vi "Test ClonSubpanel API.vi"() -> ()   [LabVIEW 2024]
doc: "ClonSubpanel API Tester."
uses:
  <vilib>/Utility/error.llb/DialogType.ctl
  ClonSubpanel.lvlib
panel:
  in  "Remove FP from Subpanel":bool
  in  "Draw FP in Supbpanel 2":bool
  in  "Draw FP in Supbpanel 1":bool
  out "last error":errorcluster
  in  "Show Diagram on Init":bool
  in  "Run as Singleton?":bool
  in  "Show Block Diagram":bool
  in  "Refresh Modules":bool
  out "Active Modules":string[](array[string])
  in  "Stop Module":bool
  in  "Select Module":i32(ring)=-1 caption="Select Module\nTo send Request to" items=["All"=-1]
  in  "Run New Module":bool
  in  "Hide Module Panel":bool
  in  "Show Module Panel":bool
  out "Status":string
  # "This VI tests the API for the Module."
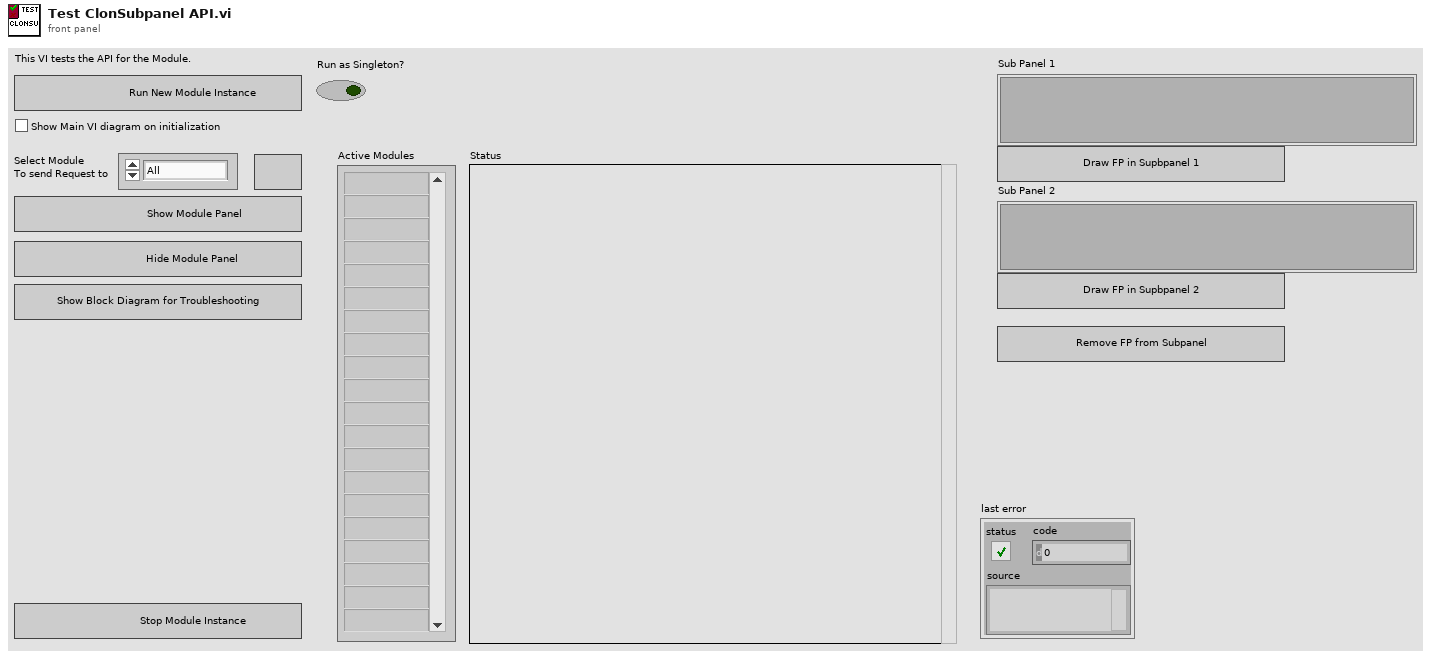
[diagram p1: front panel]
types:
  T1 = typedef "ClonSubpanel.lvlib/Broadcast Events--cluster.ctl" = cluster{"Module Did Init":refnum<user-event>, "Status Updated":refnum<user-event>, "Error Reported":refnum<user-event>, "Module Did Stop":refnum<user-event>, "Update Module Execution Status":refnum<user-event>}
  T2 = typedef "DialogType.ctl" = u16
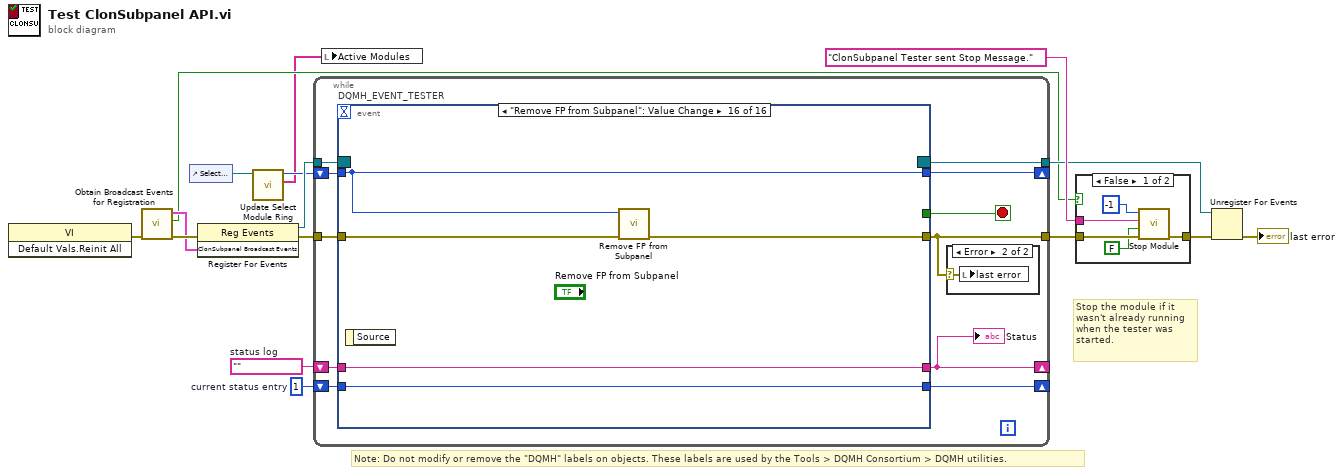
[diagram p0: block diagram]
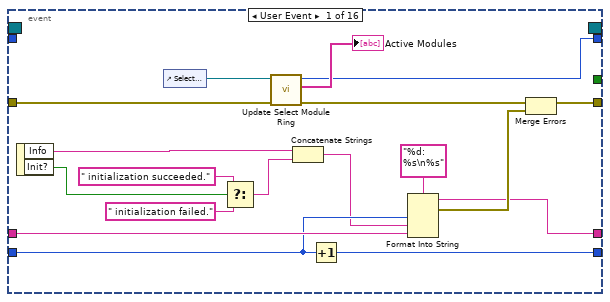
[diagram p4: hidden frame]
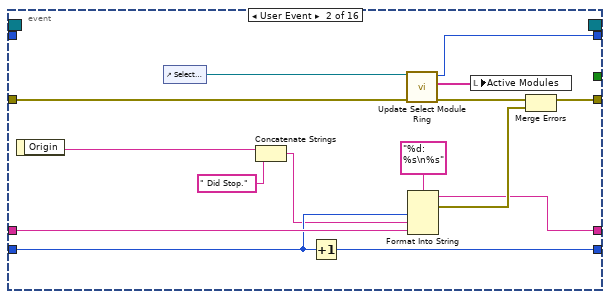
[diagram p5: hidden frame]
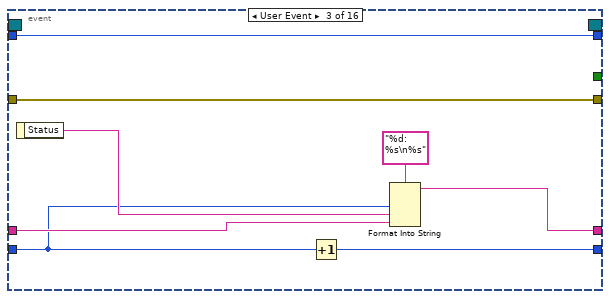
[diagram p6: hidden frame]
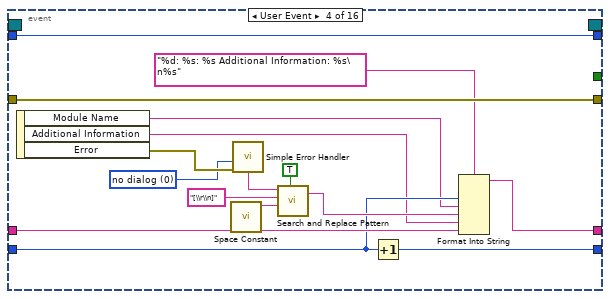
[diagram p7: hidden frame]
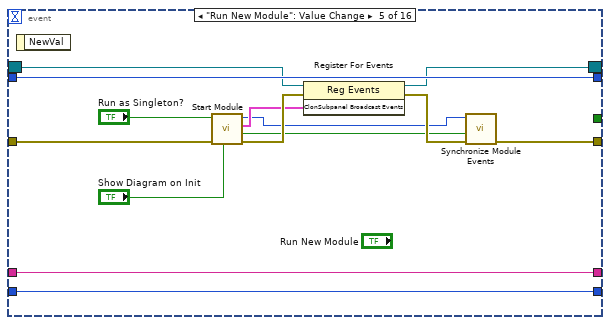
[diagram p8: hidden frame]
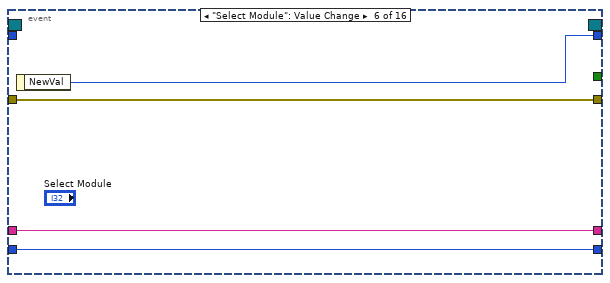
[diagram p9: hidden frame]
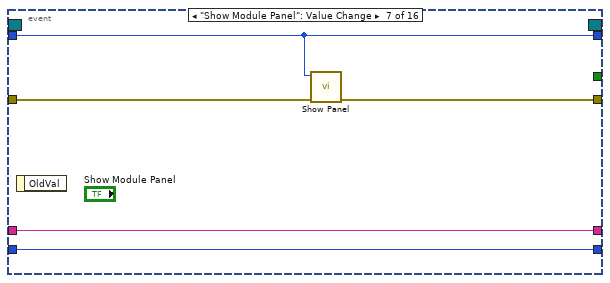
[diagram p10: hidden frame]
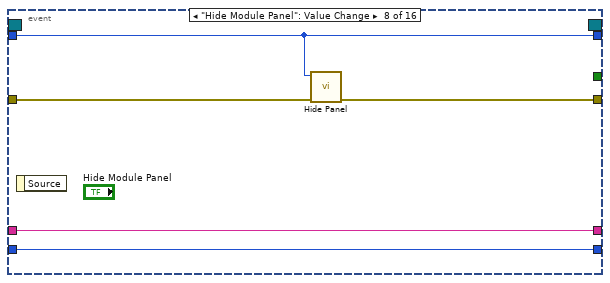
[diagram p11: hidden frame]
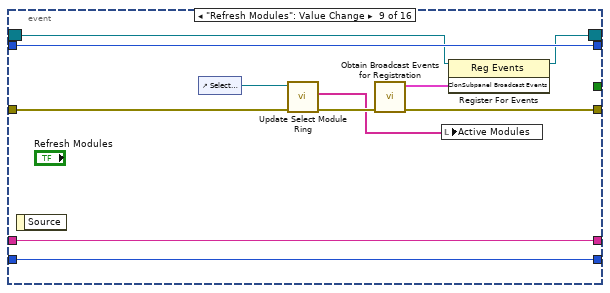
[diagram p12: hidden frame]
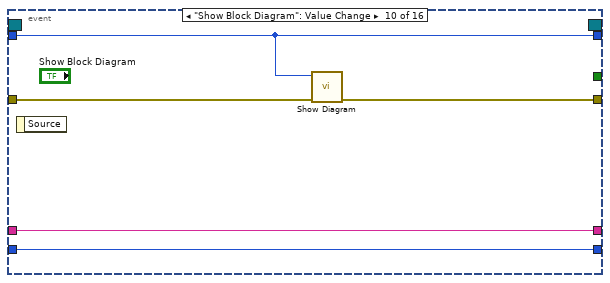
[diagram p13: hidden frame]
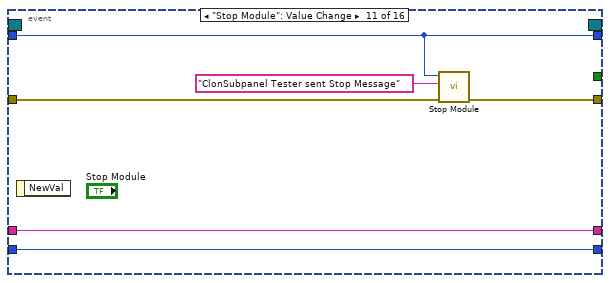
[diagram p14: hidden frame]
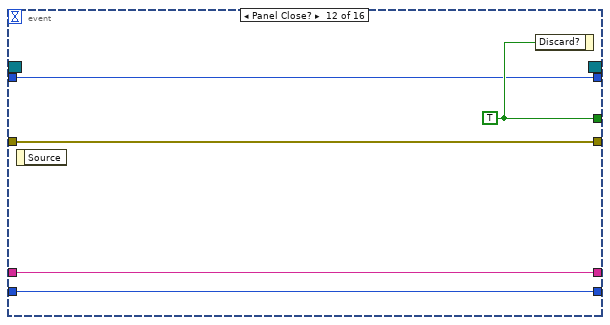
[diagram p15: hidden frame]
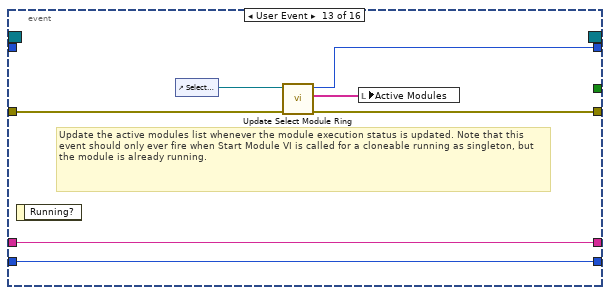
[diagram p16: hidden frame]
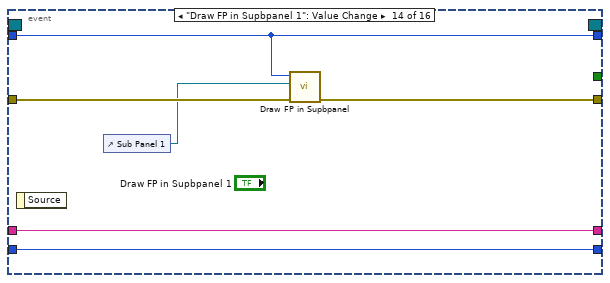
[diagram p17: hidden frame]
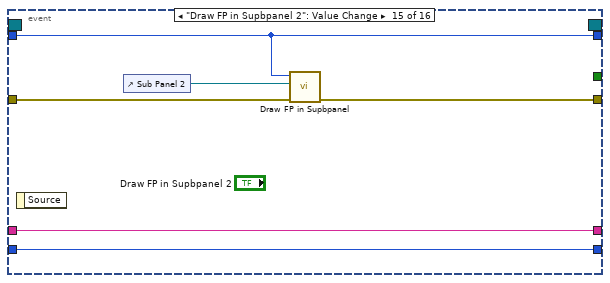
[diagram p18: hidden frame]
diagram:
  w8 = 1  # current status entry
  w9 = ""  # status log
  # "Stop the module if it wasn't already running when the tester was started."
  # "Note: Do not modify or remove the \"DQMH\" labels on objects. These labels are used by the Tools > DQMH Consortium > DQMH utilities."
  n1 = invoke class="VI" method="Default Vals.Reinit All"() -> (error out=w14:errorcluster)  [unwired: 3 in, 2 out]
  n2 = call "Obtain Broadcast Events for Registration.vi"("error in"=w14) -> ("error out"=w13:errorcluster, "Already running?"=w4:bool, "ClonSubpanel Broadcast Events"=w7:T1)  [unwired: 8 in]
  n3 = control-ref of="Select Module"() -> (w3:refnum<vi>)
  n4 = register-events(error in=w13, w7) -> (reference out=w10:refnum<event-registration>, error out=w15:errorcluster)  [unwired: 1 in]
  n5 = call "Update Select Module Ring.vi"("Select Module Ring Ref"=w3) -> ("Active Modules (Array)"=w1:string[], "New Module Ring Value"=w2:i32)  [unwired: 8 in, 1 out]
  n6 = while {
    tunnel: w10 -> [w25]
    tunnel: [w26] -> w12
    tunnel: w15 -> [w27]
    shift-right: [w21] -> _
    shift-left: w9 -> [w23]
    shift-right: [w22] -> _
    shift-left: w8 -> [w24]
    shift-right: [w19] -> _
    shift-left: w2 -> [w20]
    tunnel: [w18] -> w5
    stop <- w17 stop-if-true
    n7 = event "DQMH_EVENT_TESTER" shown="[15] \"Remove FP from Subpanel\": Value Change" {
      selector: w25 -> [_ _ _ _ w92 _ _ _ w117 _ _ _ _ _ _ _]
      dyn-events: [_ _ _ _ w91 _ _ _ w116 _ _ _ _ _ _ _] -> w18
      timeout: _ -> [_ _ _ _ _ _ _ _ _ _ _ _ _ _ _ _]
      tunnel: [_ _ _ _ _ _ _ _ _ _ _ w139 _ _ _ _] -> w17
      tunnel: [w43 w58 w69 w85 w96 w103 w107 w112 w122 w128 w134 w140 w146 w152 w158 w160] -> w26
      tunnel: w27 -> [w45 w60 w69 w85 w97 w103 w108 w113 w124 w129 w135 w140 w147 w153 w159 w164]
      tunnel: w24 -> [w40 w55 w62 w74 w94 w101 w105 w110 w120 w126 w132 w137 w144 w150 w156 w162]
      tunnel: w23 -> [w41 w56 w65 w75 w95 w102 w106 w111 w121 w127 w133 w138 w145 w151 w157 w163]
      tunnel: [w38 w53 w66 w73 w95 w102 w106 w111 w121 w127 w133 w138 w145 w151 w157 w163] -> w21
      tunnel: [w39 w54 w68 w72 w94 w101 w105 w110 w120 w126 w132 w137 w144 w150 w156 w162] -> w22
      tunnel: w20 -> [_ _ w63 w83 w93 _ w104 w109 w119 w125 w131 w136 _ w149 w155 w161]
      tunnel: [w33 w50 w63 w83 w93 w100 w104 w109 w119 w125 w131 w136 w142 w149 w155 w161] -> w19
      event User Event {
        n8 = event-data() -> ("Info"=w37:string, "Init?"=w30:bool)  [unwired: 1 in]
        n9 = control-ref of="Select Module"() -> (w35:refnum<vi>)
        n10 = Select(t=" initialization succeeded.", s=w30, f=" initialization failed.") -> (s? t:f=w29:string)
        n11 = call "Update Select Module Ring.vi"("error in"=w45, "Select Module Ring Ref"=w35) -> ("error out"=w44:errorcluster, "Active Modules (Array)"=→"Active Modules":string[], "New Module Ring Value"=w33:i32)  [unwired: 7 in]
        n12 = Concatenate Strings(w37, w29) -> (w36:string)
        n13 = Increment(x=w40) -> (x+1=w39:i32)
        n14 = Format Into String(format string="%d: %s\n%s", w40, w36, w41) -> (resulting string=w38:string, error out=w46:errorcluster)  [unwired: 2 in]
        n15 = Merge Errors(w44, w46) -> (w43:errorcluster)
      }
      event User Event {
        n16 = event-data() -> ("Origin"=w48:string)  [unwired: 1 in]
        n17 = control-ref of="Select Module"() -> (w52:refnum<vi>)
        n18 = Concatenate Strings(w48, " Did Stop.") -> (w47:string)
        n19 = Increment(x=w55) -> (x+1=w54:i32)
        n20 = call "Update Select Module Ring.vi"("error in"=w60, "Select Module Ring Ref"=w52) -> ("error out"=w59:errorcluster, "Active Modules (Array)"=w51:string[], "New Module Ring Value"=w50:i32)  [unwired: 7 in]
        n21 = Format Into String(format string="%d: %s\n%s", w55, w47, w56) -> (resulting string=w53:string, error out=w61:errorcluster)  [unwired: 2 in]
        n22 = local write "Active Modules"(w51) -> ()
        n23 = Merge Errors(w59, w61) -> (w58:errorcluster)
      }
      event User Event {
        n24 = event-data() -> ("Status"=w64:string)  [unwired: 1 in]
        n25 = Increment(x=w62) -> (x+1=w68:i32)
        n26 = Format Into String(format string="%d: %s\n%s", w62, w64, w65) -> (resulting string=w66:string)  [unwired: 2 in, 1 out]
      }
      event User Event {
        w76 = T2 0 items=["no dialog", "OK message", "continue or stop message", "OK message + warnings", "continue/stop + warnings"] ("type of dialog (OK msg:1)")
        n27 = event-data() -> ("Module Name"=w71:string, "Additional Information"=w70:string, "Error"=w84:errorcluster)  [unwired: 1 in]
        n28 = call <vilib>:"Space Constant.vi"() -> ("String"=w80:string)
        n29 = call <vilib>:"Simple Error Handler.vi"("type of dialog (OK msg:1)"=w76, "error in (no error)"=w84) -> ("message"=w77:string)  [unwired: 3 in, 4 out]
        n30 = call <vilib>:"Search and Replace Pattern.vi"("string"=w77, "regular expression (\"\")"="[\\r\\n]" ("regular expression (\"\")"), "replace string (\"\")"=w80, "replace all? (F)"=TRUE ("replace all CR/LF with spaces")) -> ("result string"=w78:string)  [unwired: 1 in, 1 out]
        n31 = Increment(x=w74) -> (x+1=w72:i32)
        n32 = Format Into String(format string="%d: %s: %s Additional Information: %s\n%s", w74, w71, w78, w70, w75) -> (resulting string=w73:string)  [unwired: 2 in, 1 out]
      }
      event "Run New Module": Value Change {
        n33 = event-data() -> ()  [unwired: 1 in, 1 out]
        n34 = call "Start Module.vi"("Show Main VI Diagram on Init (F)"="Show Diagram on Init", "error in"=w97, "Run as Singleton? (F)"="Run as Singleton?") -> ("error out"=w98:errorcluster, "Wait for Event Sync?"=w90:bool, "ClonSubpanel Broadcast Events"=w89:T1, "Module ID"=w86:i32)  [unwired: 4 in, 1 out]
        n35 = register-events(reference=w92, error in=w98, w89) -> (reference out=w91:refnum<event-registration>, error out=w99:errorcluster)
        n36 = call "Synchronize Module Events.vi"("error in"=w99, "Wait for Event Sync?"=w90, "Module ID in"=w86) -> ("error out"=w96:errorcluster)  [unwired: 7 in, 1 out]
      }
      event "Select Module": Value Change {
        n37 = event-data() -> ("NewVal"=w100:i32)  [unwired: 1 in]
      }
      event "Show Module Panel": Value Change {
        n38 = event-data() -> ()  [unwired: 1 in, 1 out]
        n39 = call "Show Panel.vi"("error in"=w108, "Module ID"=w104) -> ("error out"=w107:errorcluster)  [unwired: 9 in]
      }
      event "Hide Module Panel": Value Change {
        n40 = event-data() -> ()  [unwired: 1 in, 1 out]
        n41 = call "Hide Panel.vi"("error in"=w113, "Module ID"=w109) -> ("error out"=w112:errorcluster)  [unwired: 9 in]
      }
      event "Refresh Modules": Value Change {
        n42 = event-data() -> ()  [unwired: 1 in, 1 out]
        n43 = control-ref of="Select Module"() -> (w118:refnum<vi>)
        n44 = call "Update Select Module Ring.vi"("error in"=w124, "Select Module Ring Ref"=w118) -> ("error out"=w123:errorcluster, "Active Modules (Array)"=w114:string[])  [unwired: 7 in, 1 out]
        n45 = call "Obtain Broadcast Events for Registration.vi"("error in"=w123) -> ("error out"=w122:errorcluster, "ClonSubpanel Broadcast Events"=w115:T1)  [unwired: 8 in, 1 out]
        n46 = local write "Active Modules"(w114) -> ()
        n47 = register-events(reference=w117, w115) -> (reference out=w116:refnum<event-registration>)  [unwired: 1 in, 1 out]
      }
      event "Show Block Diagram": Value Change {
        n48 = event-data() -> ()  [unwired: 1 in, 1 out]
        n49 = call "Show Diagram.vi"("error in"=w129, "Module ID"=w125) -> ("error out"=w128:errorcluster)  [unwired: 9 in]
      }
      event "Stop Module": Value Change {
        n50 = event-data() -> ()  [unwired: 1 in, 1 out]
        n51 = call "Stop Module.vi"("error in"=w135, "Origin"="ClonSubpanel Tester sent Stop Message", "Module ID"=w131) -> ("error out"=w134:errorcluster)  [unwired: 8 in]
      }
      event Panel Close? {
        w139 = TRUE ("Discard?")
        n52 = event-data() -> ()  [unwired: 1 in, 1 out]
        n53 = event-data("Discard?"=w139) -> ()  [unwired: 1 in, 1 out]
      }
      event User Event {
        # "Update the active modules list whenever the module execution status is updated. Note that this event should only ever fire when Start Module VI is called for a cloneable running as singleton, but the module is already running."
        n54 = event-data() -> ()  [unwired: 1 in, 1 out]
        n55 = control-ref of="Select Module"() -> (w143:refnum<vi>)
        n56 = call "Update Select Module Ring.vi"("error in"=w147, "Select Module Ring Ref"=w143) -> ("error out"=w146:errorcluster, "Active Modules (Array)"=w141:string[], "New Module Ring Value"=w142:i32)  [unwired: 7 in]
        n57 = local write "Active Modules"(w141) -> ()
      }
      event "Draw FP in Supbpanel 1": Value Change {
        n58 = event-data() -> ()  [unwired: 1 in, 1 out]
        n59 = control-ref of="Sub Panel 1"() -> (w148:refnum<vi>)
        n60 = call "Draw FP in Supbpanel.vi"("error in"=w153, "Sub Panel"=w148, "Module ID"=w149) -> ("error out"=w152:errorcluster)  [unwired: 8 in]
      }
      event "Draw FP in Supbpanel 2": Value Change {
        n61 = event-data() -> ()  [unwired: 1 in, 1 out]
        n62 = control-ref of="Sub Panel 2"() -> (w154:refnum<vi>)
        n63 = call "Draw FP in Supbpanel.vi"("error in"=w159, "Sub Panel"=w154, "Module ID"=w155) -> ("error out"=w158:errorcluster)  [unwired: 8 in]
      }
      event "Remove FP from Subpanel": Value Change {
        n64 = event-data() -> ()  [unwired: 1 in, 1 out]
        n65 = call "Remove FP from Subpanel.vi"("error in"=w164, "Module ID"=w161) -> ("error out"=w160:errorcluster)  [unwired: 9 in]
      }
    }
    "Status" <- w21
    n66 = case shown="Error" w26 {
      selector: w26 -> [_ w28]
      frame No Error {
      }
      frame Error {
        n67 = local write "last error"(w28) -> ()
      }
    }
  }
  n68 = local write "Active Modules"(w1) -> ()
  n69 = case shown="False" w4 {
    tunnel: [w169 w170] -> w16
    tunnel: "ClonSubpanel Tester sent Stop Message." ("Origin") -> [w167 _]
    tunnel: w12 -> [w168 w170]
    frame False {
      n70 = call "Stop Module.vi"("error in"=w168, "Wait for Module to stop? (F)"=FALSE ("Wait for Module to stop?"), "Origin"=w167, "Module ID"=-1 ("Stop all")) -> ("error out"=w169:errorcluster)  [unwired: 7 in]
    }
    frame True {
    }
  }
  n71 = Unregister For Events(event registration refnum=w5, error in=w16) -> (error out=→"last error":errorcluster)
